vi "Untitled 1.vi"() -> ()   [LabVIEW 2015]
panel:
  out "Resultante":dbl
  in  "Valor":dbl
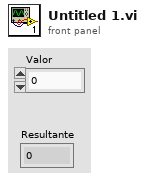
[diagram p1: front panel]
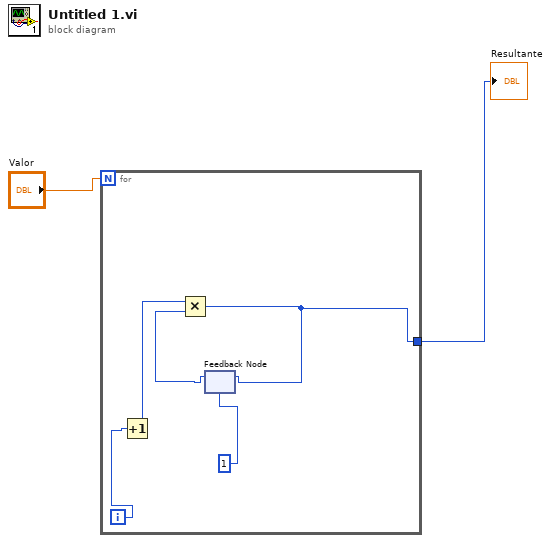
[diagram p0: block diagram]
diagram:
  n1 = for {
    N: "Valor" -> [_]
    tunnel: [w3] -> w1
    i -> [w7]
    n2 = Increment(x=w7) -> (x+1=w6:i32)
    n3 = feedback #1(1) -> (w4:i32)
    n4 = Multiply(x=w6, y=w4) -> (x*y=w3:i32)
    n5 = feedback-in #1(w3) -> ()
  }
  "Resultante" <- w1
